vi "XBEE Tx Serial Frame Processor.vi"(6 "stop":bool, 9 "TX Frame Queue":refnum<queue>, 11 "VISA Serial Port":refnum<visa-resource-name>) -> (0 "Producer error out":errorcluster, 1 "Consumer error out":errorcluster)   [LabVIEW 2016]
uses:
  WiFi API Frame Type.ctl
  WiFi API Frame.ctl
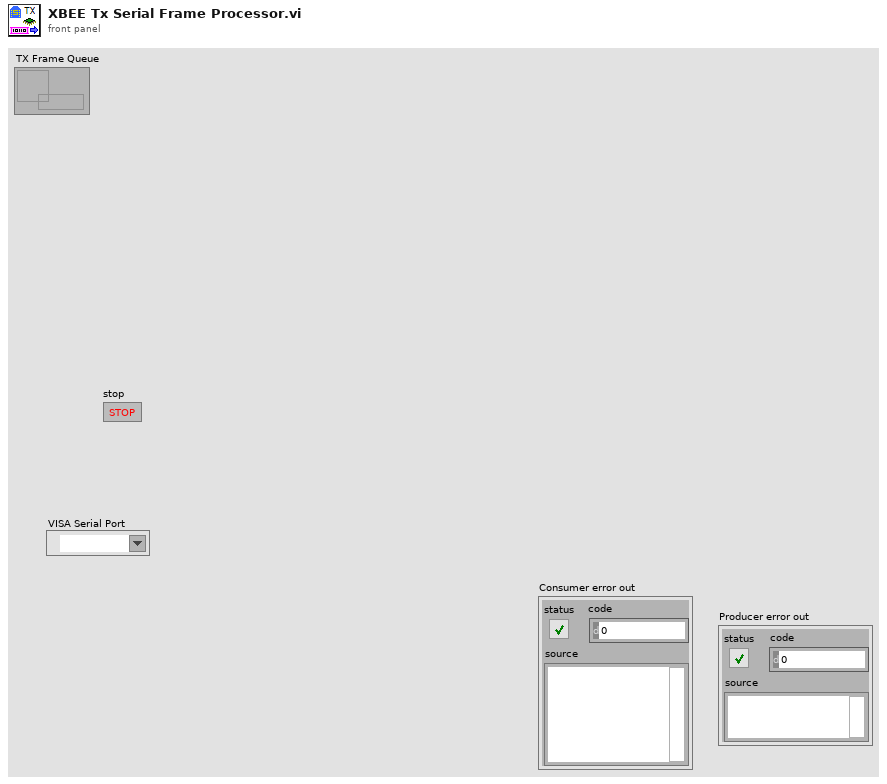
[diagram p1: front panel]
types:
  T1 = typedef "WiFi API Frame.ctl" = cluster{"Length":u16, "Frame Type":T2, "Payload":u8[], "Checksum":u8}
  T2 = typedef "WiFi API Frame Type.ctl" = u8
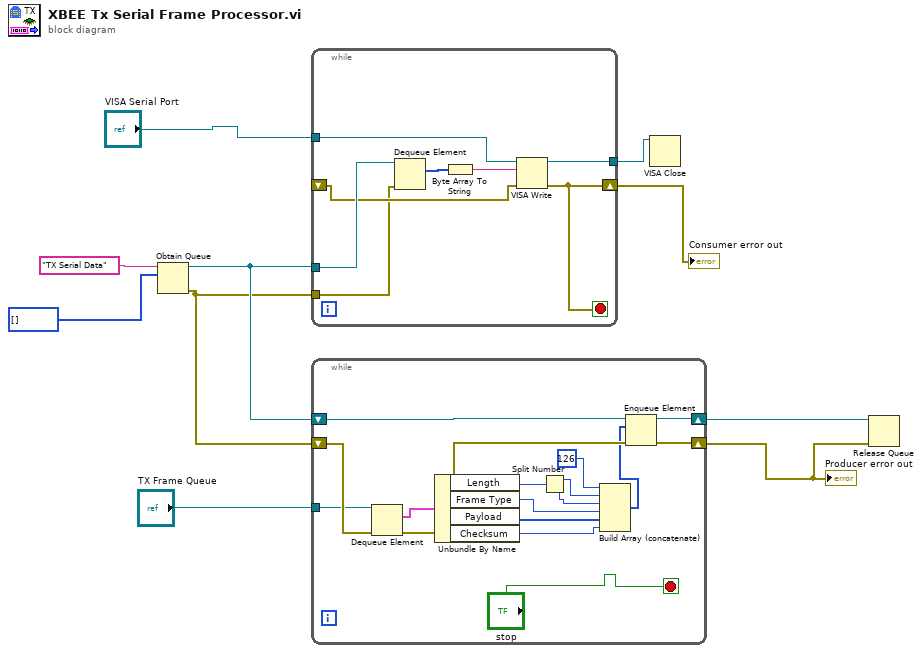
[diagram p0: block diagram]
diagram:
  n1 = Obtain Queue(name (unnamed)="TX Serial Data", element data type=u8[] []) -> (queue out=w8:refnum<queue>, error out=w4:errorcluster)  [unwired: 3 in, 1 out]
  n2 = while {
    tunnel: "VISA Serial Port" -> [w17]
    tunnel: w8 -> [w18]
    shift-right: [w12] -> w6
    shift-left: _ -> [w16]
    tunnel: [w15] -> w2
    tunnel: w4 -> [w14]
    stop <- w12 stop-if-true
    n3 = Dequeue Element(queue=w18, error in (no error)=w14) -> (element=w13:u8[])  [unwired: 1 in, 3 out]
    n4 = Byte Array To String(unsigned byte array=w13) -> (string=w11:string)
    n5 = VISA Write(VISA resource name=w17, write buffer=w11, error in (no error)=w16) -> (VISA resource name out=w15:refnum<visa-resource-name>, error out=w12:errorcluster)  [unwired: 1 out]
  }
  "Consumer error out" <- w6
  n6 = while {
    shift-right: [w31] -> w7
    shift-left: w8 -> [w34]
    shift-right: [w30] -> w5
    shift-left: w4 -> [w32]
    tunnel: "TX Frame Queue" -> [w20]
    stop <- "stop" stop-if-true
    n7 = Dequeue Element(queue=w20, error in (no error)=w32) -> (element=w19:T1, error out=w33:errorcluster)  [unwired: 1 in, 2 out]
    n8 = Unbundle By Name(w19) -> ("Length"=w29:u16, "Frame Type"=w26:T2, "Payload"=w25:u8[], "Checksum"=w24:u8)
    n9 = Split Number(x=w29) -> (hi(x)=w28:u8, lo(x)=w27:u8)
    n10 = Build Array (concatenate)(u8 126, w28, w27, w26, w25, w24) -> (w23:T2[])
    n11 = Enqueue Element(queue=w34, element=w23, error in (no error)=w33) -> (queue out=w31:refnum<queue>, error out=w30:errorcluster)  [unwired: 1 in, 1 out]
  }
  "Producer error out" <- w5
  n12 = VISA Close(VISA resource name=w2) -> ()  [unwired: 1 in, 1 out]
  n13 = Release Queue(queue=w7, error in (no error)=w5) -> ()  [unwired: 1 in, 3 out]
